vi "Create DataTable.vi"(6 "visible (false)":bool=TRUE, 8 "error in (no error)":errorcluster, 10 "table name":string, 11 "JMP application":refnum<k7>) -> (0 "error out":errorcluster, 2 "new DataTable":refnum<k7>, 3 "JMP application out":refnum<k7>)   [LabVIEW 2019, in "JMP Automation.lvlib"]
doc: "create a new DataTable\n\nJMP application: valide JMP application handle\nvisible (false): if true the table will be visible\ntable name: name of the table"
uses:
  <instrlib>/LV_JMP_bridge/JMP Automation.lvlib
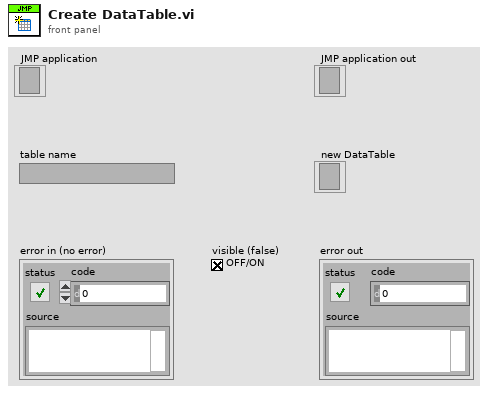
[diagram p1: front panel]
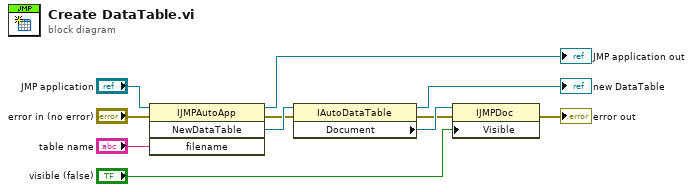
[diagram p0: block diagram]
diagram:
  n1 = invoke class="IJMPAutoApp" method="NewDataTable"(reference="JMP application", error in="error in (no error)", "filename"="table name") -> (reference out=→"JMP application out":refnum<k7>, error out=w6:errorcluster, "NewDataTable"=w7:refnum<k7>)  [unwired: 1 in, 1 out]
  n2 = property class="IAutoDataTable"(reference=w7, error in=w6) -> (reference out=→"new DataTable":refnum<k7>, error out=w2:errorcluster, "Document"=w4:refnum<k7>)
  n3 = property class="IJMPDoc"(reference=w4, error in=w2, "Visible"="visible (false)") -> (error out=→"error out":errorcluster)  [unwired: 1 out]
